vi "Set Acquisition Regs.vi"(0 "acq in":refnum<class "niUSRP Rx DSP v2 FPGA.lvclass">, 5 "dsp":T1 caption="misc") -> (4 "acq out":refnum<class "niUSRP Rx DSP v2 FPGA.lvclass">)   [LabVIEW 2025, in "niUSRP Rx DSP v2 FPGA.lvclass"]
doc: "this VI is an Acquisition class accessor for private data."
uses:
  niUSRP Rx DSP v2 FPGA.lvclass
  Typedefs/DSP Shared Regs.ctl
  niUSRP Rx DSP v2 FPGA.lvclass/niUSRP Rx DSP v2 FPGA.ctl
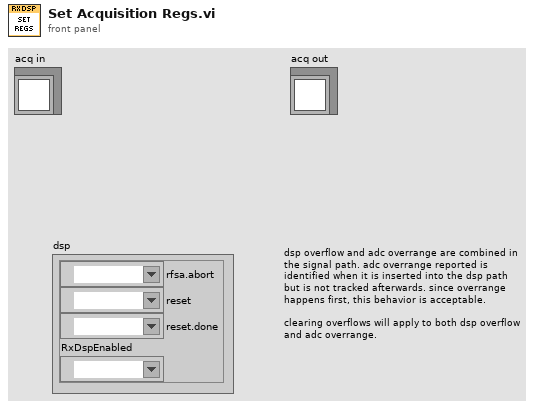
[diagram p1: front panel]
types:
  T1 = typedef "niUSRP Rx DSP v2 FPGA.lvclass/DSP Shared Regs.ctl" = cluster{"rfsa.abort":refnum<k21>, "reset":refnum<k21>, "reset.done":refnum<k21>, "RxDspEnabled":refnum<k21>}
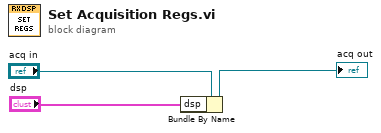
[diagram p0: block diagram]
diagram:
  n1 = Bundle By Name(cluster="acq in", "dsp"="dsp") -> (→"acq out":refnum<class "niUSRP Rx DSP v2 FPGA.lvclass">)
